vi "Open Connection.vi"(8 "error in (no error)":errorcluster) -> (0 "error out":errorcluster, 3 "connection ID":refnum<k5>)   [LabVIEW 2013, in "libssh2_integration_tests.lvlib"]
uses:
  libssh2_integration_tests.lvlib
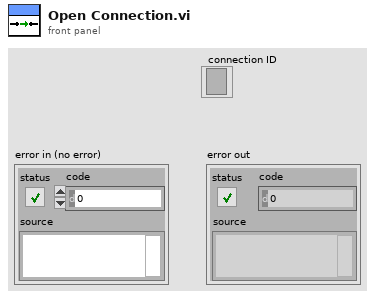
[diagram p1: front panel]
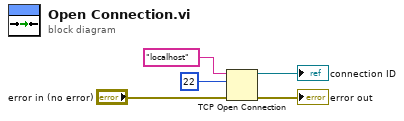
[diagram p0: block diagram]
diagram:
  n1 = TCP Open Connection(address="localhost", remote port or service name=u16 22, error in (no error)="error in (no error)") -> (connection ID=→"connection ID":refnum<k5>, error out=→"error out":errorcluster)  [unwired: 2 in]
